vi "测试.vi"() -> ()   [LabVIEW 2020]
uses:
  Lib/2601B/2601B.lvclass
  8649b9f9-8ffd-41c6-913b-8276f7b27aa5.vi
  6d43c680-a1f8-4723-bf79-b62a09ce1ae1.vi
  viLib/LogLib/LogLib.lvlib
  viLib/QueueLib/QueueLib.lvlib
  D:/Workspace/LabVIEW/MemristorCharacterization/Lib/2601B/2601B.lvclass
panel:
  out "触发按钮":T1(tab)
  in  "扫描负":bool
  in  "扫描正":bool
  in  "循环":bool
  out "剩余":u32
  in  "次数":u32=1 min=1 max=100
  in  "保持时间":bool
  in  "脉冲2":bool
  in  "脉冲1":bool
  in  "高速脉冲1":bool
  in  "高速脉冲2":bool
  in  "任意波形":bool
  in  "功能选择":T2(xcontrol)
  in  "删除":bool
  in  "样品标记":string(combo)
  in  "停止":bool
  in  "数据显示":dbl[][](xcontrol)
  out "测试人员":string
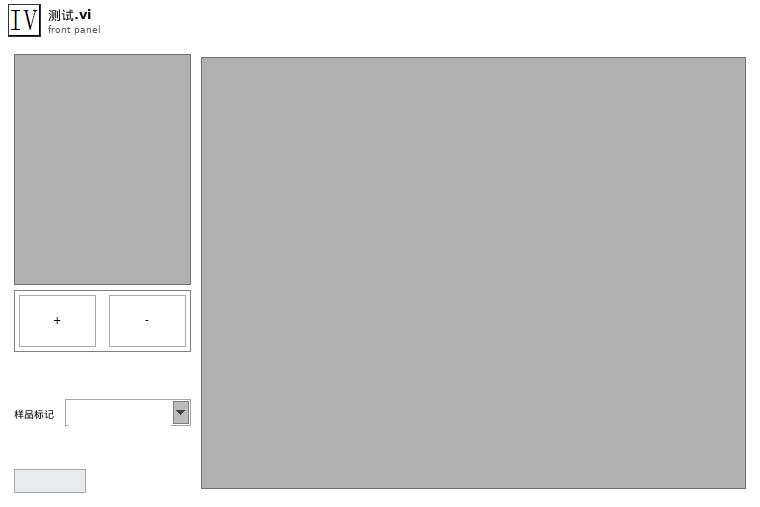
[diagram p1: front panel]
types:
  T1 = enum32{"扫描", "循环扫描", "保持时间", "脉冲", "高速脉冲", "任意波形"}
  T2 = enum16{"扫描", "循环扫描", "保持时间", "脉冲", "高速脉冲", "任意波形"}
  T3 = typedef "队列组.ctl" = cluster{"2601B":refnum<queue>, "数据处理":refnum<queue>}
  T4 = typedef "功能选择.xctl/方向属性.ctl" = enum16{"1", "2"}
  T5 = enum8{"Enabled", "Disabled", "Disabled and Grayed Out"}
  T6 = typedef "QueueLib.lvlib/数据类型.ctl" = cluster{"消息":string, "数据":variant}
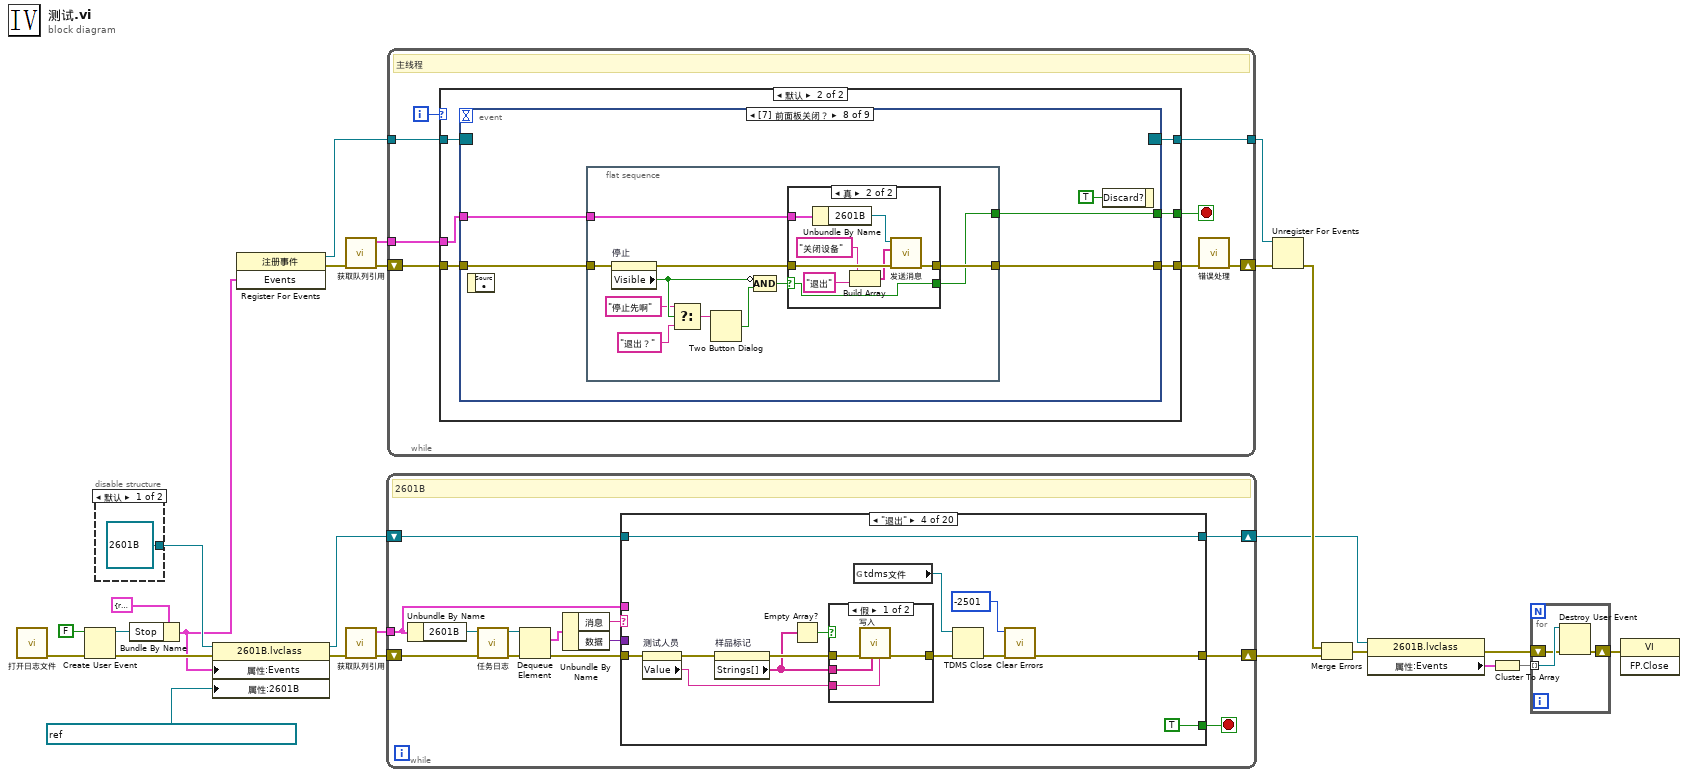
[diagram p0: block diagram]
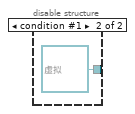
[diagram p2: hidden frame]
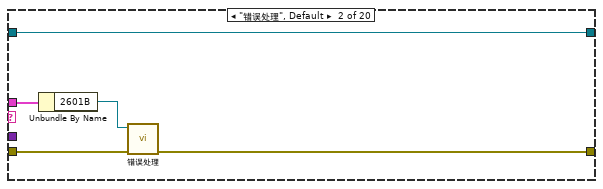
[diagram p4: hidden frame]
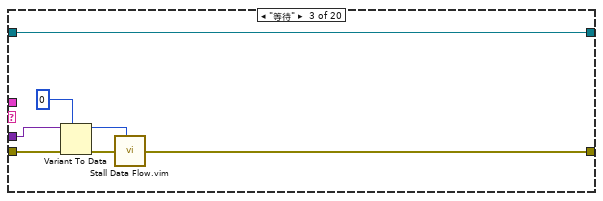
[diagram p5: hidden frame]
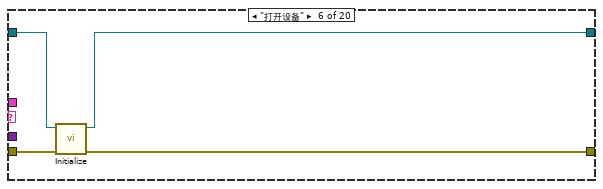
[diagram p8: hidden frame]
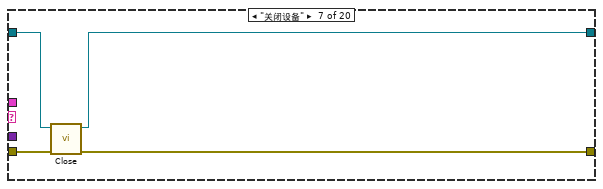
[diagram p9: hidden frame]
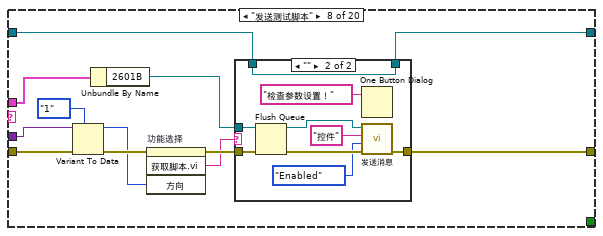
[diagram p10: hidden frame]
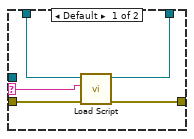
[diagram p11: hidden frame]
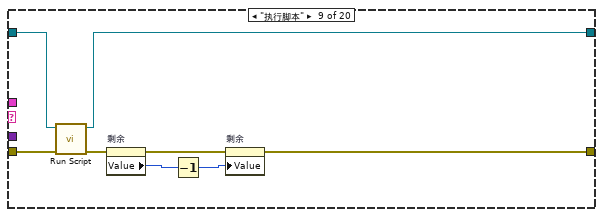
[diagram p12: hidden frame]
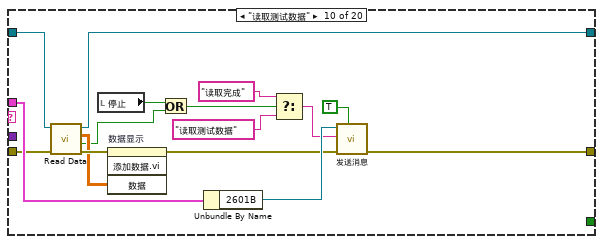
[diagram p13: hidden frame]
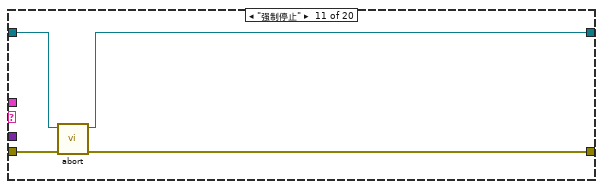
[diagram p14: hidden frame]
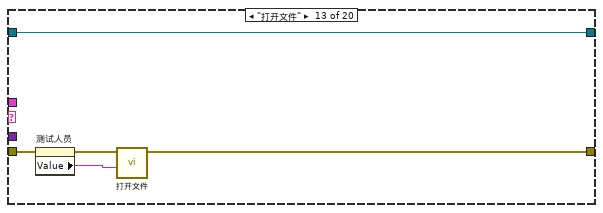
[diagram p16: hidden frame]
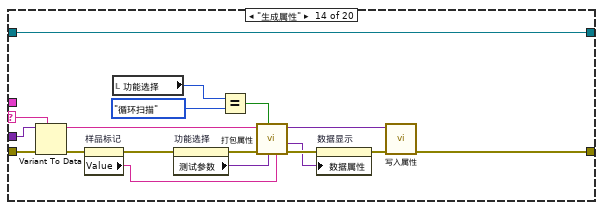
[diagram p17: hidden frame]
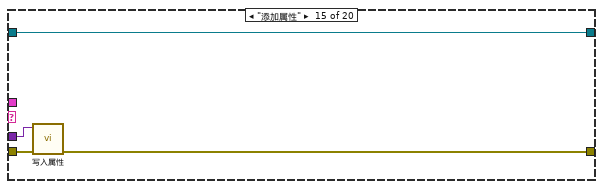
[diagram p18: hidden frame]
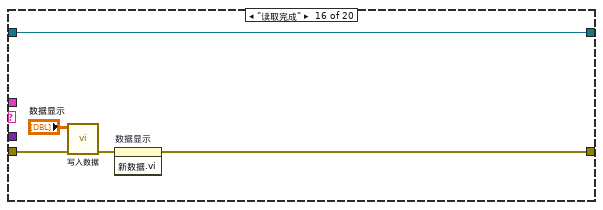
[diagram p19: hidden frame]
diagram:
  n1 = call "打开日志文件.vi"() -> ("错误输出"=w2:errorcluster)  [unwired: 11 in]
  n2 = Create User Event(user event datatype=FALSE ("事件数据"), error in=w2) -> (user event=w19:refnum<user-event>, error out=w15:errorcluster)
  n3 = disable-structure shown="默认" {
    disable-tunnel: [refnum<class "2601B.lvclass"> refnum ("2601B.lvclass") refnum<class "虚拟.lvclass"> refnum ("虚拟.lvclass")] -> w22
    frame condition #0 (active) {
    }
    frame condition #1 {
    }
  }
  n4 = Bundle By Name(cluster=cluster{"Stop":refnum<user-event>} {"Stop"=refnum} ("Events"), "Stop"=w19) -> (w14:cluster{"Stop":refnum<user-event>})
  n5 = property class="2601B.lvclass"(reference=w22, error in=w15, "属性:Events"=w14, "属性:2601B"=refnum<visa-resource-name> "USB0::0x05E6::0x2601::4469244::INSTR" ("2601B")) -> (reference out=w16:refnum<class "2601B.lvclass">, error out=w17:errorcluster)
  n6 = register-events(w14) -> (reference out=w13:refnum<event-registration>, error out=w1:errorcluster)  [unwired: 2 in]
  n7 = call "获取队列引用.vi"("错误输入（无错误）"=w1) -> ("错误输出"=w25:errorcluster, "队列组"=w26:T3)  [unwired: 9 in]
  n8 = call "获取队列引用.vi"("错误输入（无错误）"=w17) -> ("错误输出"=w23:errorcluster, "队列组"=w24:T3)  [unwired: 9 in]
  n9 = while {
    tunnel: w24 -> [w36]
    shift-right: [w37] -> w10
    shift-left: w23 -> [w35]
    shift-right: [w29] -> w7
    shift-left: w16 -> [w30]
    stop <- w31 stop-if-true
    # "2601B"
    n10 = Unbundle By Name(w36) -> ("2601B"=w33:refnum<queue>)
    n11 = call "任务日志.vi"("错误输入（无错误）"=w35, "队列输入"=w33) -> ("错误输出"=w34:errorcluster, "队列输出"=w32:refnum<queue>)  [unwired: 8 in]
    n12 = Dequeue Element(queue=w32, error in (no error)=w34) -> (element=w41:T6, error out=w40:errorcluster)  [unwired: 1 in, 2 out]
    n13 = Unbundle By Name(w41) -> ("消息"=w39:string, "数据"=w38:variant)
    n14 = case shown="\"退出\"" w39 {
      selector: w39 -> [_ _ _ _ _ _ _ _ _ _ _ _ _ w159 _ _ _ _ _ _]
      tunnel: [w43 w47 w52 w59 w75 w79 w82 w86 w114 w128 w136 w139 w140 w148 w164 w167 w173 w179 w185 w202] -> w37
      tunnel: w40 -> [w43 w48 w55 w61 w75 w78 w83 w94 w112 w132 w137 w139 w141 w162 w166 w168 w173 w178 w186 w201]
      tunnel: w38 -> [_ _ w53 _ _ _ _ w95 _ _ _ _ _ w160 w163 _ _ _ _ w199]
      tunnel: w36 -> [_ w46 _ _ _ _ _ w89 _ w133 _ _ _ _ _ _ _ _ _ _]
      tunnel: [_ _ _ TRUE ("事件数据") _ _ _ _ _ _ _ _ _ _ _ _ _ _ _ _] -> w31
      tunnel: w30 -> [w42 w44 w49 w60 w74 w77 w80 w85 w111 w130 w134 w138 w144 w151 w165 w171 w172 w180 w187 w191]
      tunnel: [w42 w44 w49 w60 w74 w76 w81 w84 w110 w131 w135 w138 w144 w151 w165 w171 w172 w180 w187 w191] -> w29
      frame "==== 标准任务 ====" {
      }
      frame "错误处理", Default {
        n15 = Unbundle By Name(w46) -> ("2601B"=w45:refnum<queue>)
        n16 = call "错误处理.vi"("错误输入（无错误）"=w48, "队列输入"=w45) -> ("错误输出"=w47:errorcluster)  [unwired: 8 in, 1 out]
      }
      frame "等待" {
        n17 = Variant To Data(error in=w55, type=u32 0 ("milliseconds to wait"), Variant=w53) -> (data=w50:u32, error out=w54:errorcluster)
        n18 = call "Stall Data Flow.vim"("value in"=w54, "milliseconds to wait"=w50) -> ("value out"=w52:errorcluster)  [unwired: 1 out]
      }
      frame "退出" {
        n19 = property on="测试人员" class="Str"(error in=w61) -> (error out=w67:errorcluster, "Value"=w65:string)  [unwired: 1 in, 1 out]
        n20 = property on="样品标记" class="CmbBox"(error in=w67) -> (error out=w68:errorcluster, "Strings[]"=w56:string[])  [unwired: 1 in, 1 out]
        n21 = Empty Array?(array=w56) -> (empty?=w57:bool)
        n22 = case shown="假" w57 {
          tunnel: w68 -> [w72 w73]
          tunnel: [w71 w73] -> w66
          tunnel: w65 -> [w70 _]
          tunnel: w56 -> [w69 _]
          frame False {
            n23 = call "写入.vi"("测试人员"=w70, "样品标记"=w69, "error in (no error)"=w72) -> ("error out"=w71:errorcluster)  [unwired: 8 in]
          }
          frame True {
          }
        }
        n24 = global read "TDMS引用.vi" "tdms文件"() -> (w64:refnum<k34>)
        n25 = TDMS Close(8:w66, 11:w64) -> (0:w63:errorcluster)  [unwired: 1 out]
        n26 = call <vilib>:"Clear Errors.vi"("error in (no error)"=w63, "specific error code to clear (0: all)"=-2501) -> ("error out"=w59:errorcluster)  [unwired: 4 in, 1 out]
      }
      frame "==== 2601B ====" {
      }
      frame "打开设备" {
        n27 = call-dynamic "Initialize.vi"("error in (no error)"=w78, "2601B 输入"=w77) -> ("error out"=w79:errorcluster, "2601B 输出"=w76:refnum<class "2601B.lvclass">)  [unwired: 8 in]
      }
      frame "关闭设备" {
        n28 = call-dynamic "Close.vi"("error in (no error)"=w83, "2601B 输入"=w80) -> ("error out"=w82:errorcluster, "2601B 输出"=w81:refnum<class "2601B.lvclass">)  [unwired: 8 in]
      }
      frame "发送测试脚本" {
        n29 = Variant To Data(error in=w94, type=方向属性."1" ("方向"), Variant=w95) -> (data=w91:T4, error out=w92:errorcluster)
        n30 = Unbundle By Name(w89) -> ("2601B"=w88:refnum<queue>)
        n31 = invoke on="功能选择" class="功能选择 (严格)" method="获取脚本.vi"(error in=w92, "方向"=w91) -> (error out=w90:errorcluster, "获取脚本.vi"=w87:string)  [unwired: 2 in, 2 out]
        n32 = case shown="\"\"" w87 {
          selector: w87 -> [w96 _]
          tunnel: w90 -> [w100 w109]
          tunnel: w88 -> [_ w108]
          tunnel: [w99 w103] -> w86
          tunnel: w85 -> [w98 w101]
          tunnel: [w97 w101] -> w84
          frame Default {
            n33 = call-dynamic "Load Script.vi"("error in (no error)"=w100, "Script"=w96, "2601B 输入"=w98) -> ("error out"=w99:errorcluster, "2601B 输出"=w97:refnum<class "2601B.lvclass">)  [unwired: 7 in]
          }
          frame "" {
            n34 = Flush Queue(queue=w108, error in (no error)=w109) -> (queue out=w106:refnum<queue>, error out=w107:errorcluster)  [unwired: 1 out]
            n35 = One Button Dialog(message="检查参数设置！" ("消息")) -> ()  [unwired: 1 in, 1 out]
            n36 = call-poly "发送消息.vi"("错误输入（无错误）"=w107, "数据"=T5."Enabled" ("禁用"), "消息"="控件", "输入队列"=w106) -> ("错误输出"=w103:errorcluster)  [unwired: 6 in, 1 out]
          }
        }
      }
      frame "执行脚本" {
        n37 = call-dynamic "Run Script.vi"("error in (no error)"=w112, "2601B 输入"=w111) -> ("error out"=w113:errorcluster, "2601B 输出"=w110:refnum<class "2601B.lvclass">)  [unwired: 8 in]
        n38 = property on="剩余" class="DigNum (严格)"(error in=w113) -> (error out=w115:errorcluster, "Value"=w116:u32)  [unwired: 1 in, 1 out]
        n39 = Decrement(x=w116) -> (x-1=w117:u32)
        n40 = property on="剩余" class="DigNum (严格)"(error in=w115, "Value"=w117) -> (error out=w114:errorcluster)  [unwired: 1 in, 1 out]
      }
      frame "读取测试数据" {
        n41 = call-dynamic "Read Data.vi"("error in (no error)"=w132, "2601B 输入"=w130) -> ("error out"=w126:errorcluster, "完成"=w119:bool, "DBL"=w121:dbl[][], "2601B 输出"=w131:refnum<class "2601B.lvclass">)  [unwired: 6 in]
        n42 = local read "停止"() -> (w120:bool)
        n43 = invoke on="数据显示" class="数据显示 (严格)" method="添加数据.vi"(error in=w126, "数据"=w121) -> (error out=w125:errorcluster)  [unwired: 2 in, 3 out]
        n44 = Or(x=w120, y=w119) -> (x .or. y?=w118:bool)
        n45 = Unbundle By Name(w133) -> ("2601B"=w129:refnum<queue>)
        n46 = Select(t="读取完成" ("消息"), s=w118, f="读取测试数据" ("消息")) -> (s? t:f=w122:string)
        n47 = call-poly "发送消息.vi"("强制优先"=TRUE, "错误输入（无错误）"=w125, "消息"=w122, "输入队列"=w129) -> ("错误输出"=w128:errorcluster)  [unwired: 6 in, 1 out]
      }
      frame "强制停止" {
        n48 = call-dynamic "abort.vi"("error in (no error)"=w137, "2601B 输入"=w134) -> ("error out"=w136:errorcluster, "2601B 输出"=w135:refnum<class "2601B.lvclass">)  [unwired: 8 in]
      }
      frame "==== 数据 ====" {
      }
      frame "打开文件" {
        n49 = property on="测试人员" class="Str"(error in=w141) -> (error out=w143:errorcluster, "Value"=w142:string)  [unwired: 1 in, 1 out]
        n50 = call "打开文件.vi"("测试人员"=w142, "错误输入（无错误）"=w143) -> ("错误输出"=w140:errorcluster)  [unwired: 9 in]
      }
      frame "生成属性" {
        n51 = Variant To Data(error in=w162, type=w159, Variant=w160) -> (data=w155:string, error out=w161:errorcluster)
        n52 = property on="样品标记" class="CmbBox"(error in=w161) -> (error out=w157:errorcluster, "Value"=w158:string)  [unwired: 1 in, 1 out]
        n53 = local read "功能选择"() -> (w154:T2)
        n54 = property on="功能选择" class="功能选择 (严格)"(error in=w157) -> (error out=w156:errorcluster, "测试参数"=w147:variant)  [unwired: 1 in, 1 out]
        n55 = Equal?(x=w154, y=T2."循环扫描") -> (x = y?=w152:bool)
        n56 = call "打包属性.vi"("样品标记"=w158, "测试参数"=w147, "循环"=w152, "错误输入"=w156, "功能"=w155) -> ("错误输出"=w150:errorcluster, "测试参数输出"=w145:variant, "数据属性"=w149:variant)  [unwired: 4 in]
        n57 = property on="数据显示" class="数据显示 (严格)"(error in=w150, "数据属性"=w145) -> (error out=w146:errorcluster)  [unwired: 1 in, 1 out]
        n58 = call "写入属性.vi"("错误输入（无错误）"=w146, "数据属性"=w149) -> ("错误输出"=w148:errorcluster)  [unwired: 9 in]
      }
      frame "添加属性" {
        n59 = call "写入属性.vi"("错误输入（无错误）"=w166, "数据属性"=w163) -> ("错误输出"=w164:errorcluster)  [unwired: 9 in]
      }
      frame "读取完成" {
        n60 = call "写入数据.vi"("错误输入（无错误）"=w168, "测试数据"="数据显示") -> ("错误输出"=w169:errorcluster)  [unwired: 9 in]
        n61 = invoke on="数据显示" class="数据显示 (严格)" method="新数据.vi"(error in=w169) -> (error out=w167:errorcluster)  [unwired: 2 in, 2 out]
      }
      frame "==== 用户界面 ====" {
      }
      frame "用户名" {
        n62 = call "输入用户名"("error in (no error)"=w178) -> ("用户名"=w177:string, "error out"=w179:errorcluster)  [unwired: 16 in, 1 out]
        n63 = Empty String/Path?(string/path=w177) -> (empty?=w175:bool)
        n64 = Select(t="Default", s=w175, f=w177) -> (s? t:f=→"测试人员":string)
      }
      frame "读取样品标记" {
        n65 = property on="测试人员" class="Str"(error in=w186) -> (error out=w183:errorcluster, "Value"=w184:string)  [unwired: 1 in, 1 out]
        n66 = call "读取.vi"("测试人员"=w184, "error in (no error)"=w183) -> ("error out"=w182:errorcluster, "样品标记"=w181:string[])  [unwired: 8 in]
        n67 = property on="样品标记" class="CmbBox"(error in=w182, "Strings[]"=w181) -> (error out=w185:errorcluster)  [unwired: 1 in, 1 out]
      }
      frame "控件" {
        w192 = T5."Enabled" ("禁用")
        n68 = Variant To Data(error in=w201, type=w192, Variant=w199) -> (data=w193:T5, error out=w200:errorcluster)
        n69 = Not Equal?(x=w193, y=w192) -> (x != y?=w189:bool)
        n70 = property on="停止" class="Bool (严格)"(error in=w200, "Visible"=w189, "Value"=FALSE ("停止")) -> (error out=w196:errorcluster)  [unwired: 1 in, 1 out]
        n71 = property on="剩余" class="DigNum (严格)"(error in=w196, "Visible"=w189) -> (error out=w195:errorcluster)  [unwired: 1 in, 1 out]
        n72 = Not(x=w189) -> (.not. x?=w188:bool)
        n73 = property on="删除" class="Bool"(error in=w195, "Visible"=w188) -> (error out=w190:errorcluster)  [unwired: 1 in, 1 out]
        n74 = control-ref of="本VI"() -> (w198:refnum<vi>)
        n75 = call "禁用控件.vi"("控件名称"=string[] ["功能选择", "触发按钮", "样品标记"], "本VI"=w198, "错误输入（无错误）"=w190, "禁用"=w193) -> ("错误输出"=w202:errorcluster)  [unwired: 7 in]
      }
    }
  }
  n76 = while {
    tunnel: w26 -> [w208]
    shift-right: [w205] -> w12
    shift-left: w25 -> [w209]
    tunnel: w13 -> [w204]
    tunnel: [w203] -> w11
    i -> [w210]
    stop <- w207 stop-if-true
    # "主线程"
    n77 = case shown="默认" w210 {
      tunnel: w209 -> [w213 w229]
      tunnel: [w212 w227] -> w206
      tunnel: w208 -> [w214 w228]
      tunnel: [_ w225] -> w207
      tunnel: w204 -> [w211 w226]
      tunnel: [w211 w224] -> w203
      frame 0 {
        n78 = flat-sequence {
          tunnel: w214 -> [w223]
          tunnel: w213 -> [w222]
          tunnel: [w217] -> w212
          frame #0 {
            n79 = Unbundle By Name(w223) -> ("2601B"=w221:refnum<queue>)
            n80 = call-poly "发送消息.vi"("错误输入（无错误）"=w222, "消息"="打开设备", "输入队列"=w221) -> ("错误输出"=w218:errorcluster)  [unwired: 7 in, 1 out]
            n81 = control-ref of="本VI"() -> (w219:refnum<vi>)
            n82 = call "禁用控件.vi"("控件名称"=string[] ["功能选择", "触发按钮", "样品标记", "数据显示", "测试人员"], "本VI"=w219, "错误输入（无错误）"=w218, "禁用"=T5."Disabled and Grayed Out") -> ("错误输出"=w217:errorcluster)  [unwired: 7 in]
          }
        }
      }
      frame Default {
        n83 = event shown="[7] 前面板关闭？" {
          selector: w226 -> [_ _ _ _ _ _ _ _ _]
          dyn-events: [_ _ _ _ _ _ _ _ _] -> w224
          timeout: _ -> [_ _ _ _ _ _ _ _ _]
          tunnel: w229 -> [w231 w253 w260 w284 w305 w315 w330 w345 w372]
          tunnel: [w233 w252 w257 w283 w307 w316 w328 w346 w371] -> w227
          tunnel: w228 -> [_ _ w258 w282 w306 w317 w329 w347 w370]
          tunnel: [_ _ _ _ _ _ _ w344 w369] -> w225
          event "样品标记": Value Change {
            n84 = event-data() -> ("NewVal"=w230:string, "OldVal"=w232:string)  [unwired: 1 in]
            n85 = flat-sequence {
              tunnel: [w236] -> w233
              tunnel: w230 -> [w241]
              tunnel: w232 -> [w240]
              tunnel: w231 -> [w237]
              frame #0 {
                n86 = property on="样品标记" class="CmbBox"(error in=w237) -> (error out=w235:errorcluster, "Strings[]"=w239:string[])  [unwired: 1 in, 1 out]
                n87 = case shown="\"\"" w241 {
                  selector: w241 -> [w243 _]
                  tunnel: w240 -> [_ w248]
                  tunnel: w239 -> [w246 w251]
                  tunnel: [w244 w249] -> w238
                  tunnel: w235 -> [w242 w247]
                  tunnel: [w242 w247] -> w234
                  frame Default {
                    n88 = Build Array (concatenate)(w246, w243) -> (w245:string[])
                    n89 = call "Remove Duplicates From 1D Array.vim"("array"=w245) -> ("array with duplicates removed"=w244:string[])  [unwired: 10 in]
                  }
                  frame "" {
                    n90 = Search 1D Array(1D array=w251, element=w248) -> (index of element=w250:i32)  [unwired: 1 in]
                    n91 = Delete From Array(array=w251, index=w250) -> (array with subset deleted=w249:string[])  [unwired: 1 in, 1 out]
                  }
                }
                n92 = property on="样品标记" class="CmbBox"(error in=w234, "Strings[]"=w238) -> (error out=w236:errorcluster)  [unwired: 1 in, 1 out]
              }
            }
          }
          event "功能选择": Value Change {
            n93 = event-data() -> ()  [unwired: 1 in, 1 out]
            n94 = flat-sequence {
              tunnel: w253 -> [w256]
              tunnel: [w255] -> w252
              frame #0 {
                n95 = property on="数据显示" class="数据显示 (严格)"(error in=w256, "扫描"="功能选择") -> (error out=w255:errorcluster)  [unwired: 1 in, 1 out]
                "触发按钮" <- "功能选择"
              }
            }
          }
          event "扫描正", "保持时间", "脉冲1", "高速脉冲1", "任意波形": Value Change {
            n96 = event-data() -> ("CtlRef"=w259:refnum<vi>)  [unwired: 1 in]
            n97 = flat-sequence {
              tunnel: w259 -> [w279]
              tunnel: w260 -> [w278]
              tunnel: w258 -> [w265]
              tunnel: [w266] -> w261
              tunnel: [w280] -> w257
              tunnel: w261 -> [w280]
              frame #0 {
                w272 = variant
                w262 = "控件" ("消息")
                n98 = property class="Bool"(reference=w279, error in=w278) -> (error out=w267:errorcluster, "Label.Text"=w270:string)  [unwired: 1 out]
                n99 = Unbundle By Name(w265) -> ("2601B"=w264:refnum<queue>)
                n100 = Build Array(w262, "发送测试脚本" ("消息"), "生成属性" ("消息"), "执行脚本" ("消息"), "读取测试数据" ("消息"), w262) -> (w269:string[])
                n101 = Build Array(T5."Disabled and Grayed Out" ("禁用"), 方向属性."1" ("方向"), w270, w272, w272, T5."Enabled" ("禁用")) -> (w268:variant[])
                n102 = call-poly "发送消息.vi"("错误输入（无错误）"=w267, "数据列表"=w268, "消息列表"=w269, "输入队列"=w264) -> ("错误输出"=w266:errorcluster)  [unwired: 6 in, 1 out]
              }
              frame #1 {
              }
            }
          }
          event "扫描负", "脉冲2", "高速脉冲2": Value Change {
            n103 = event-data() -> ("CtlRef"=w285:refnum<vi>)  [unwired: 1 in]
            n104 = flat-sequence {
              tunnel: w285 -> [w303]
              tunnel: w284 -> [w302]
              tunnel: w282 -> [w289]
              tunnel: [w290] -> w281
              tunnel: [w304] -> w283
              tunnel: w281 -> [w304]
              frame #0 {
                w296 = variant
                w286 = "控件" ("消息")
                n105 = property class="Bool"(reference=w303, error in=w302) -> (error out=w291:errorcluster, "Label.Text"=w294:string)  [unwired: 1 out]
                n106 = Unbundle By Name(w289) -> ("2601B"=w288:refnum<queue>)
                n107 = Build Array(w286, "发送测试脚本" ("消息"), "生成属性" ("消息"), "执行脚本" ("消息"), "读取测试数据" ("消息"), w286) -> (w293:string[])
                n108 = Build Array(T5."Disabled and Grayed Out" ("禁用"), 方向属性."2" ("方向"), w294, w296, w296, T5."Enabled" ("禁用")) -> (w292:variant[])
                n109 = call-poly "发送消息.vi"("错误输入（无错误）"=w291, "数据列表"=w292, "消息列表"=w293, "输入队列"=w288) -> ("错误输出"=w290:errorcluster)  [unwired: 6 in, 1 out]
              }
              frame #1 {
              }
            }
          }
          event "循环": Value Change {
            n110 = event-data() -> ()  [unwired: 1 in, 1 out]
            n111 = flat-sequence {
              tunnel: [w311] -> w307
              tunnel: w306 -> [w310]
              tunnel: w305 -> [w308]
              frame #0 {
                n112 = Unbundle By Name(w310) -> ("2601B"=w312:refnum<queue>)
                n113 = call "生成任务队列.vi"("循环次数"="次数") -> ("任务数据"=w314:variant[], "任务名称"=w313:string[])  [unwired: 9 in]
                n114 = call-poly "发送消息.vi"("错误输入（无错误）"=w308, "数据列表"=w314, "消息列表"=w313, "输入队列"=w312) -> ("错误输出"=w311:errorcluster)  [unwired: 6 in, 1 out]
                "剩余" <- "次数"
              }
            }
          }
          event "停止": Value Change {
            n115 = event-data() -> ()  [unwired: 1 in, 1 out]
            n116 = flat-sequence {
              tunnel: w317 -> [w326]
              tunnel: [w325] -> w316
              tunnel: w315 -> [w323]
              frame #0 {
                n117 = Unbundle By Name(w326) -> ("2601B"=w327:refnum<queue>)
                n118 = Flush Queue(queue=w327, error in (no error)=w323) -> (queue out=w324:refnum<queue>, error out=w322:errorcluster)  [unwired: 1 out]
                n119 = Build Array(variant, T5."Enabled" ("禁用")) -> (w318:variant[])
                n120 = call-poly "发送消息.vi"("错误输入（无错误）"=w322, "数据列表"=w318, "消息列表"=string[] ["强制停止", "控件"], "输入队列"=w324) -> ("错误输出"=w325:errorcluster)  [unwired: 6 in, 1 out]
              }
            }
          }
          event "删除": Value Change {
            n121 = event-data() -> ()  [unwired: 1 in, 1 out]
            n122 = flat-sequence {
              tunnel: w330 -> [w335]
              tunnel: w329 -> [w340]
              tunnel: [w331] -> w328
              frame #0 {
                n123 = Unbundle By Name(w340) -> ("2601B"=w341:refnum<queue>)
                n124 = Set Variant Attribute(Variant=variant ("变体"), name="删除" ("字符串"), value=TRUE, error in=w335) -> (Variant out=w336:variant, error out=w334:errorcluster)  [unwired: 1 out]
                n125 = call-poly "发送消息.vi"("错误输入（无错误）"=w334, "数据"=w336, "消息"="添加属性", "输入队列"=w341) -> ("错误输出"=w332:errorcluster)  [unwired: 6 in, 1 out]
                n126 = property on="删除" class="Bool"(error in=w332, "Visible"=FALSE ("可见")) -> (error out=w331:errorcluster)  [unwired: 1 in, 1 out]
              }
            }
          }
          event Panel Close? {
            n127 = event-data() -> ()  [unwired: 1 in, 1 out]
            n128 = flat-sequence {
              tunnel: [w348] -> w344
              tunnel: w347 -> [w358]
              tunnel: [w357] -> w346
              tunnel: w345 -> [w356]
              frame #0 {
                n129 = property on="停止" class="Bool (严格)"(error in=w356) -> (error out=w355:errorcluster, "Visible"=w352:bool)  [unwired: 1 in, 1 out]
                n130 = Select(t="停止先啊", s=w352, f="退出？" ("消息")) -> (s? t:f=w351:string)
                n131 = Two Button Dialog(message=w351) -> (T button?=w354:bool)  [unwired: 2 in]
                n132 = Compound Arithmetic op=AND ("复合运算")(invert w352, w354) -> (w353:bool)
                n133 = case shown="真" w353 {
                  selector: w353 -> [w359 w361]
                  tunnel: w358 -> [_ w368]
                  tunnel: [w360 w366] -> w357
                  tunnel: w355 -> [w360 w365]
                  tunnel: [w359 w361] -> w348
                  frame False {
                  }
                  frame True {
                    n134 = Unbundle By Name(w368) -> ("2601B"=w367:refnum<queue>)
                    n135 = Build Array("关闭设备" ("元素"), "退出" ("消息")) -> (w363:string[])
                    n136 = call-poly "发送消息.vi"("错误输入（无错误）"=w365, "消息列表"=w363, "输入队列"=w367) -> ("错误输出"=w366:errorcluster)  [unwired: 7 in, 1 out]
                  }
                }
              }
            }
            n137 = event-data("Discard?"=TRUE ("放弃？")) -> ()  [unwired: 1 in, 1 out]
          }
          event User Event {
            n138 = event-data() -> ("布尔"=w369:bool)  [unwired: 1 in]
            n139 = case shown="假" w369 {
              tunnel: w372 -> [w384 w387]
              tunnel: [w373 w386] -> w371
              tunnel: w370 -> [w383 w385]
              frame False {
                n140 = Unbundle By Name(w383) -> ("2601B"=w382:refnum<queue>)
                n141 = Build Array("用户名", "读取样品标记" ("元素"), "打开文件" ("元素")) -> (w381:string[])
                n142 = call-poly "发送消息.vi"("错误输入（无错误）"=w384, "消息列表"=w381, "输入队列"=w382) -> ("错误输出"=w374:errorcluster)  [unwired: 7 in, 1 out]
                n143 = control-ref of="本VI"() -> (w377:refnum<vi>)
                n144 = call "禁用控件.vi"("控件名称"=string[] ["功能选择", "触发按钮", "样品标记", "数据显示", "测试人员"], "本VI"=w377, "错误输入（无错误）"=w374, "禁用"=T5."Enabled") -> ("错误输出"=w373:errorcluster)  [unwired: 7 in]
              }
              frame True {
                n145 = Unbundle By Name(w385) -> ("2601B"=w389:refnum<queue>)
                n146 = call-poly "发送消息.vi"("错误输入（无错误）"=w387, "消息"="退出", "输入队列"=w389) -> ("错误输出"=w386:errorcluster)  [unwired: 7 in, 1 out]
              }
            }
          }
        }
      }
    }
    n147 = call "错误处理.vi"("错误输入（无错误）"=w206) -> ("错误输出"=w205:errorcluster)  [unwired: 9 in, 1 out]
  }
  n148 = Unregister For Events(event registration refnum=w11, error in=w12) -> (error out=w9:errorcluster)
  n149 = Merge Errors(w9, w10) -> (w8:errorcluster)
  n150 = property class="2601B.lvclass"(reference=w7, error in=w8) -> (error out=w4:errorcluster, "属性:Events"=w6:cluster{"Stop":refnum<user-event>})  [unwired: 1 out]
  n151 = Cluster To Array(cluster=w6) -> (array=w5:refnum<user-event>[])
  n152 = for {
    tunnel: w5 -> [w392] mode=indexing
    shift-right: [w390] -> w3
    shift-left: w4 -> [w391]
    n153 = Destroy User Event(user event=w392, error in=w391) -> (error out=w390:errorcluster)
  }
  n154 = invoke class="VI" method="FP.Close"(error in=w3) -> ()  [unwired: 2 in, 3 out]
